vi "Remove-action.vi"(8 "error in (no error)":errorcluster, 11 "Object ref in":T1) -> (0 "error out":errorcluster, 3 "Object ref out":T1)   [LabVIEW 2013, in "PowderDeposition.lvlib" / "PD-Main.lvclass"]
uses:
  PD-Main.lvclass
  Object-reference.ctl
  PD-Main.lvclass/PD-Main.ctl
  Assembly/Motor-assembly.lvclass
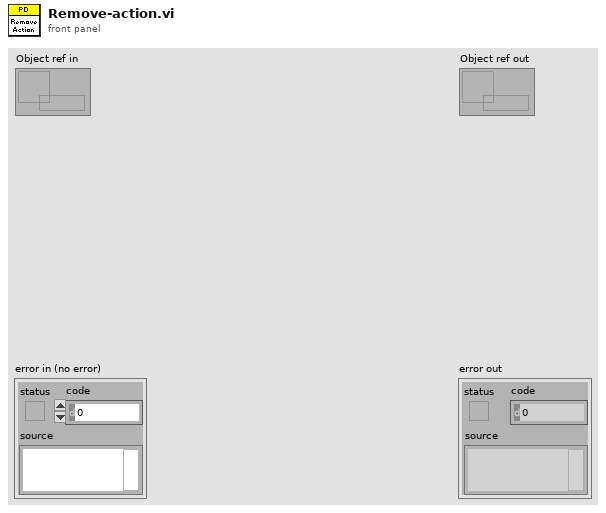
[diagram p1: front panel]
types:
  T1 = typedef "PowderDeposition.lvlib/PD-Main.lvclass/Object-reference.ctl" = refnum<data-value>
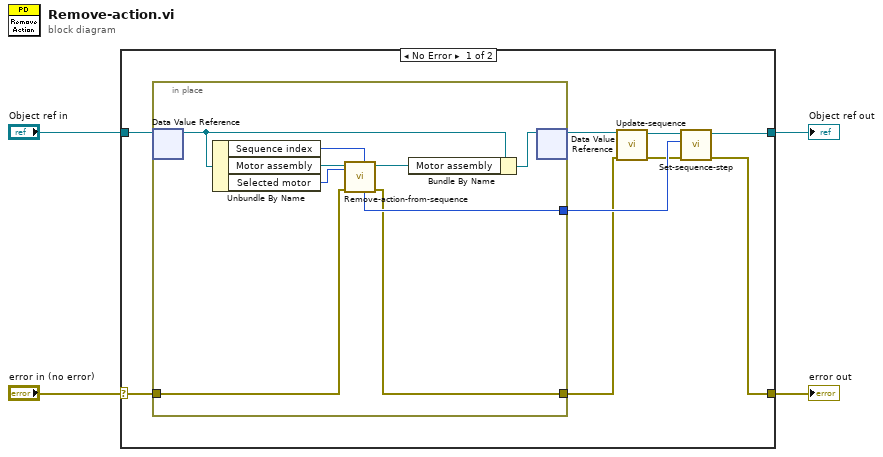
[diagram p0: block diagram]
diagram:
  n1 = case shown="No Error" "error in (no error)" {
    selector: "error in (no error)" -> [w12 w24]
    tunnel: [w10 w24] -> w3
    tunnel: [w11 w23] -> w1
    tunnel: "Object ref in" -> [w13 w23]
    frame No Error {
      n2 = in-place {
        in-place-border: [w14] -> w6
        in-place-border: w12 -> [w18]
        in-place-border: [w16] -> w9
        n3 = in-place-dvr #1(w13) -> (w22:refnum<class "PD-Main.lvclass">)  [unwired: 1 out]
        n4 = Unbundle By Name(w22) -> ("Sequence index"=w17:i32, "Motor assembly"=w20:refnum<class "Motor-assembly.lvclass">, "Selected motor"=w15:i32)
        n5 = call "Remove-action-from-sequence.vi"("Sequence index in"=w17, "Motor index"=w15, "error in (no error)"=w18, "Available motors in"=w20) -> ("error out"=w14:errorcluster, "Available motors out"=w19:refnum<class "Motor-assembly.lvclass">, "Sequence index"=w16:i32)  [unwired: 4 in, 1 out]
        n6 = Bundle By Name(cluster=w22, "Motor assembly"=w19) -> (w21:refnum<class "PD-Main.lvclass">)
        n7 = in-place-dvr #1(w21) -> (w8:T1)  [unwired: 1 out]
      }
      n8 = call "Update-sequence.vi"("error in (no error)"=w6, "Object ref in"=w8) -> ("error out"=w5:errorcluster, "Object ref out"=w7:T1)  [unwired: 8 in]
      n9 = call "Set-sequence-step.vi"("error in (no error)"=w5, "Sequence step in"=w9, "Object ref in"=w7) -> ("error out"=w10:errorcluster, "Object ref out"=w11:T1)  [unwired: 6 in, 1 out]
    }
    frame Error {
    }
  }
  "error out" <- w3
  "Object ref out" <- w1
